vi "SI 256 Grey Scale.vi"() -> (0 "?":u32[](array[numeric]))   [LabVIEW 2015]
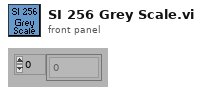
[diagram p1: front panel]
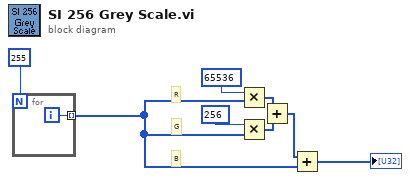
[diagram p0: block diagram]
diagram:
  # "B"
  # "G"
  # "R"
  n1 = for {
    N: 255 -> [_]
    tunnel: [w9] -> w2 mode=indexing
    i -> [w9]
  }
  n2 = Multiply(x=u32 65536, y=w2) -> (x*y=w7:u32[])
  n3 = Multiply(x=u32 256, y=w2) -> (x*y=w6:u32[])
  n4 = Add(x=w7, y=w6) -> (x+y=w8:u32[])
  n5 = Add(x=w8, y=w2) -> (x+y=→"?":u32[])
